vi "Split Array In Two.vi"(11 "array type (2D Dbl) out 3":u8[](array[numeric])) -> (2 "array type (2D Dbl) out":u8[](array[numeric]), 3 "array type (2D Dbl) out 2":u8[](array[numeric]))   [LabVIEW 2019, in "Day 6.lvlib"]
uses:
  Day 6.lvlib
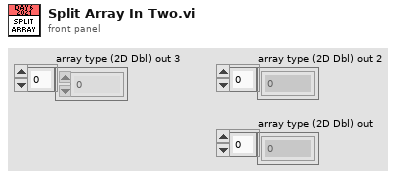
[diagram p1: front panel]
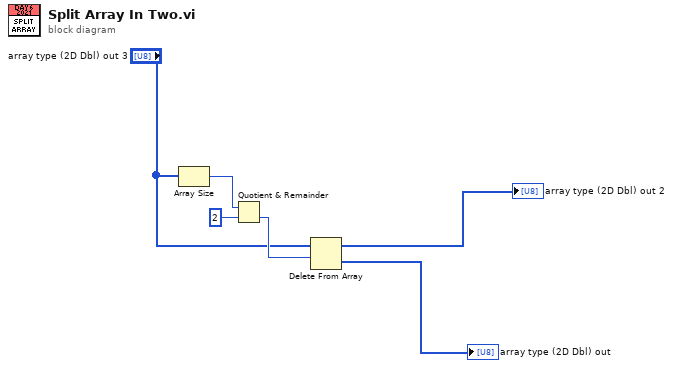
[diagram p0: block diagram]
diagram:
  n1 = Array Size(array="array type (2D Dbl) out 3") -> (size(s)=w2:i32)
  n2 = Quotient & Remainder(x=w2, y=2) -> (floor(x/y)=w4:i32)  [unwired: 1 out]
  n3 = Delete From Array(array="array type (2D Dbl) out 3", length=w4) -> (deleted portion=→"array type (2D Dbl) out":u8[], array with subset deleted=→"array type (2D Dbl) out 2":u8[])  [unwired: 1 in]
